vi "PI Controller (SubVI).vi"(0 "sp":dbl, 1 "pv":dbl, 4 "maxim":dbl, 5 "minim":dbl, 8 "p":dbl, 13 "errsum":dbl, 14 "i":dbl, 17 "h":dbl) -> (20 "output variable":dbl, 27 "errsum":dbl)   [LabVIEW 2011]
panel:
  out "integ":dbl
  out "prop":dbl
  out "err":dbl
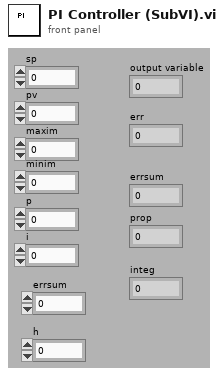
[diagram p1: front panel]
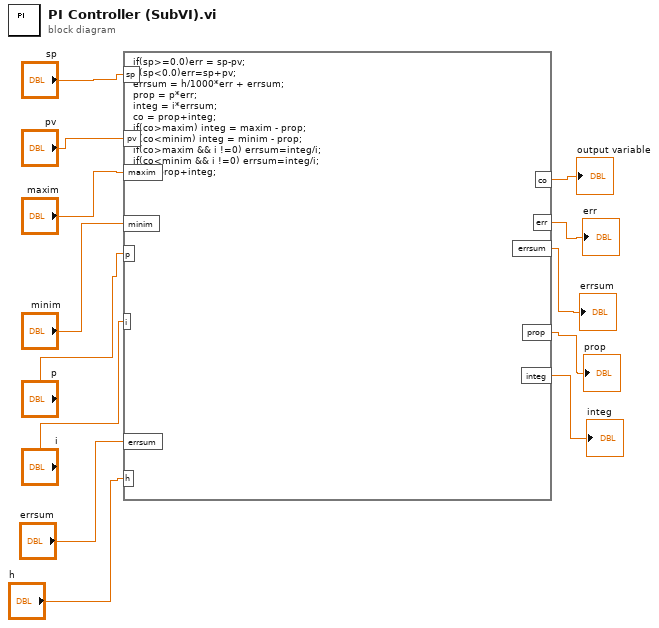
[diagram p0: block diagram]
diagram:
  n1 = formula code="if(sp>=0.0)err = sp-pv;\nif(sp<0.0)err=sp+pv;\nerrsum = h/1000*err + errsum;\nprop = p*err;\ninteg = i*errsum;\nco = prop+integ;\nif(co>maxim) integ = maxim - prop;\nif(co<minim) integ = minim - prop;\nif(co>maxim && i !=0) errsum=integ/i;\nif(co<minim && i !=0) errsum=integ/i;\nco = prop+integ;"("sp"="sp", "pv"="pv", "maxim"="maxim", "minim"="minim", "p"="p", "i"="i", "errsum"="errsum", "h"="h") -> ("co"=→"output variable":dbl, "err"=→"err":dbl, "errsum"=→"errsum":dbl, "prop"=→"prop":dbl, "integ"=→"integ":dbl)
